vi "Create New Microservice.vi"() -> ()   [LabVIEW 2019, in "MicronToolsMenu.lvlib"]
uses:
  MicronToolsMenu.lvlib
  <vilib>/Utility/error.llb/DialogType.ctl
  <vilib>/SLL Toolkit/SLL Queued State Machine/Queue Driver/Create Queue.vi
  <vilib>/SLL Toolkit/SLL Queued State Machine/Queue Driver/Enqueue an Item to Queue.vi
  <vilib>/SLL Toolkit/SLL Queued State Machine/Queue Driver/Dequeue Queue.vi
  <vilib>/SLL Toolkit/SLL Queued State Machine/Queue Driver/Enqueue N Items.vi
  <vilib>/SLL Toolkit/SLL Queued State Machine/Queue Driver/Flush Queue.vi
  <vilib>/SLL Toolkit/SLL Queued State Machine/Queue Driver/Release Queue.vi
  <vilib>/SLL Toolkit/SLL Queued State Machine/SLL QSM.lvlib
panel:
  out "Status":string
  out "New Microservice Path Output":path
  in  "New Microservice Name":string
  in  "Root Directory":path
  in  "Create":bool
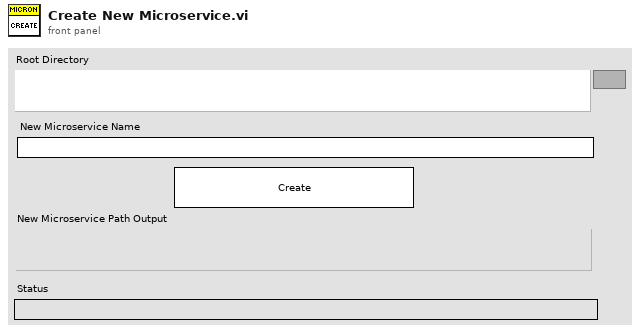
[diagram p1: front panel]
types:
  T1 = typedef "DialogType.ctl" = u16
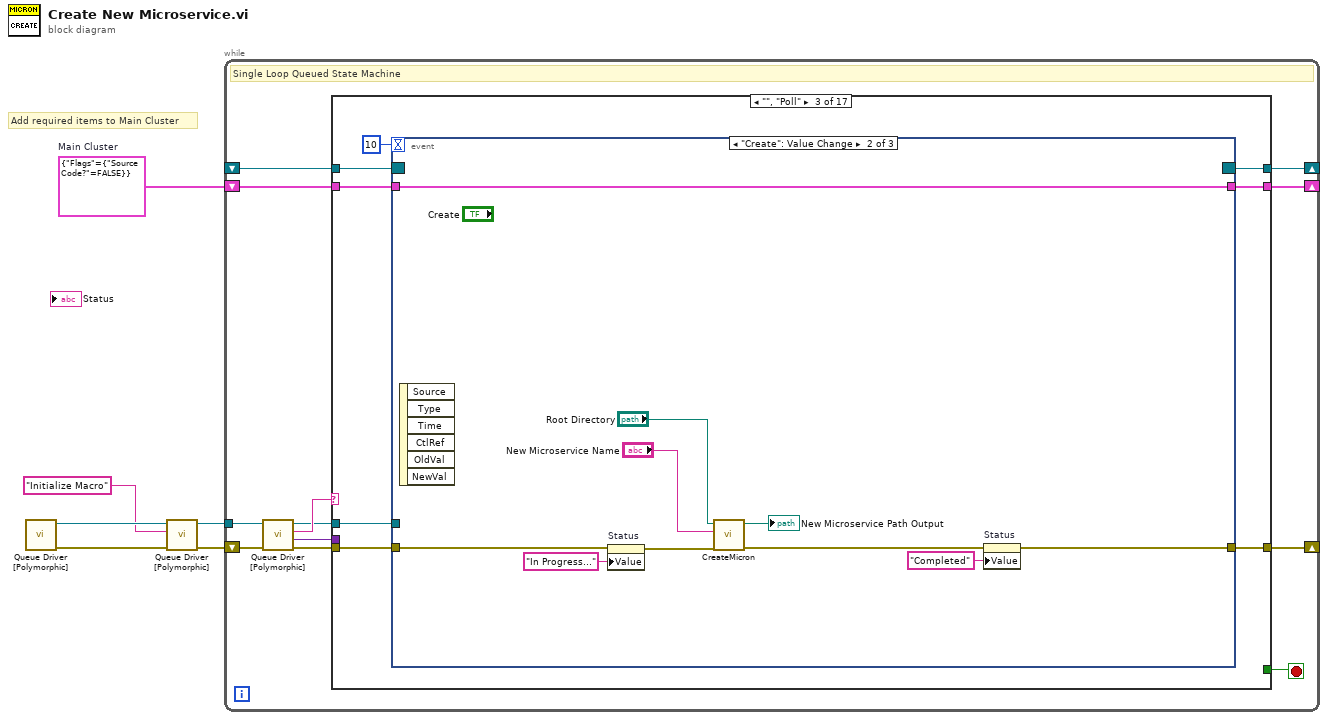
[diagram p0: block diagram]
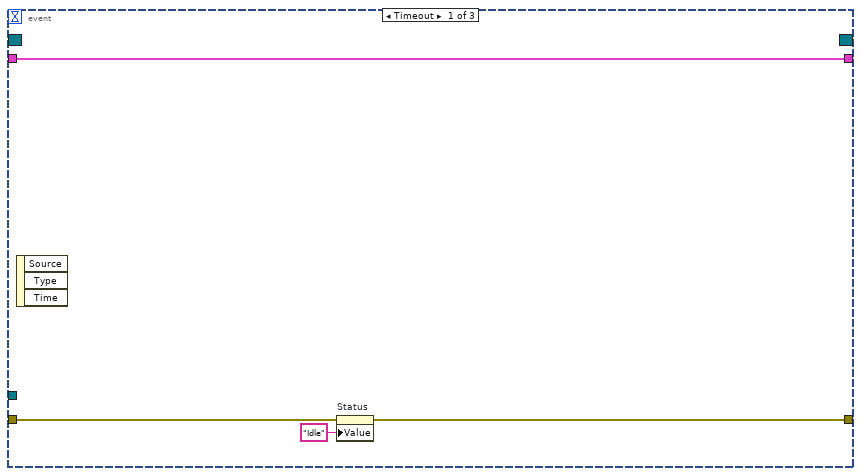
[diagram p4: hidden frame]
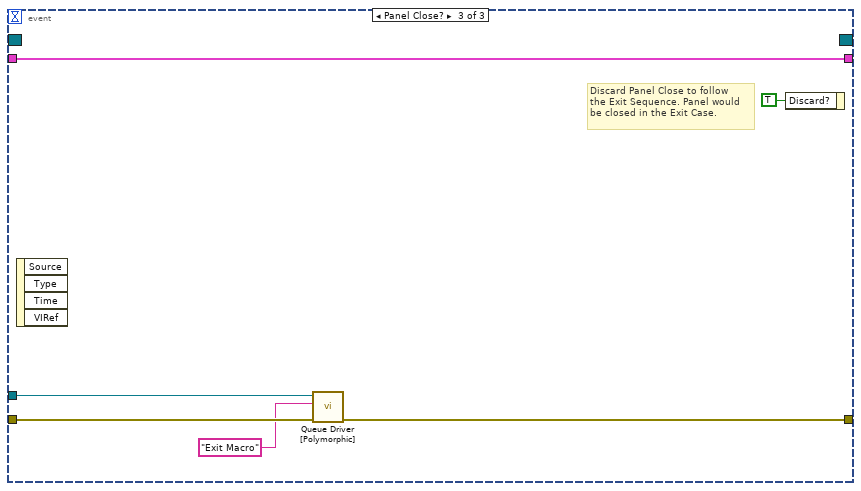
[diagram p5: hidden frame]
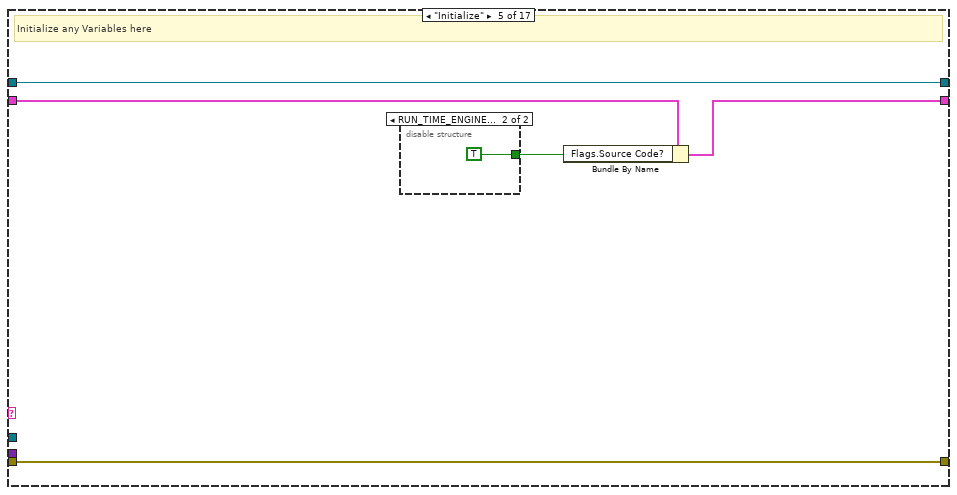
[diagram p7: hidden frame]
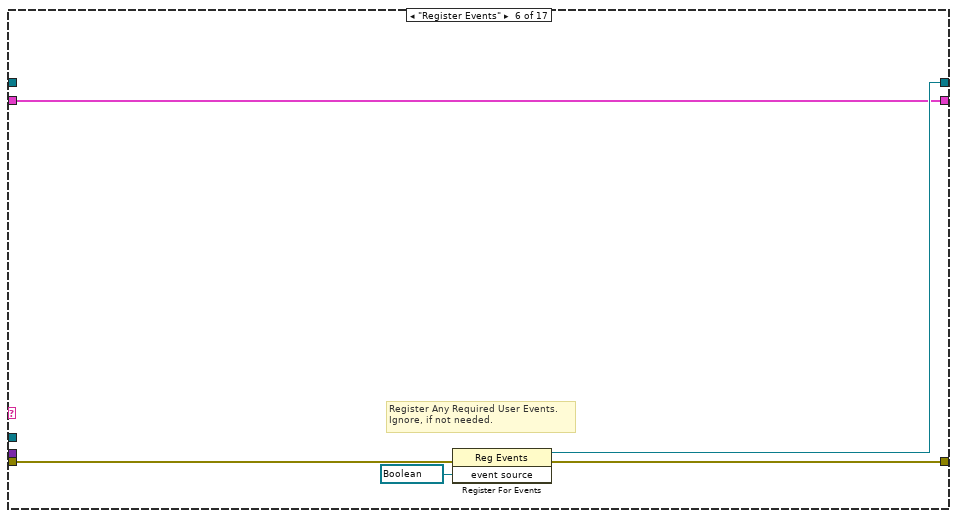
[diagram p9: hidden frame]
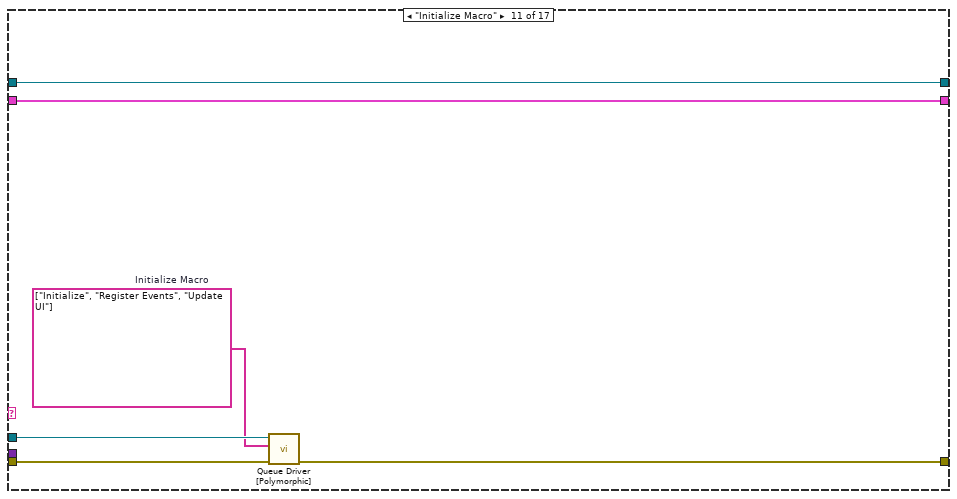
[diagram p14: hidden frame]
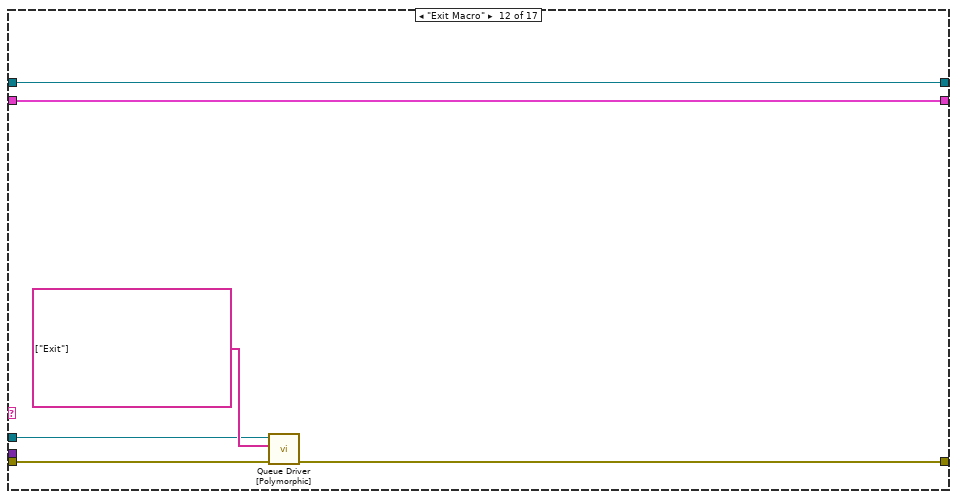
[diagram p15: hidden frame]
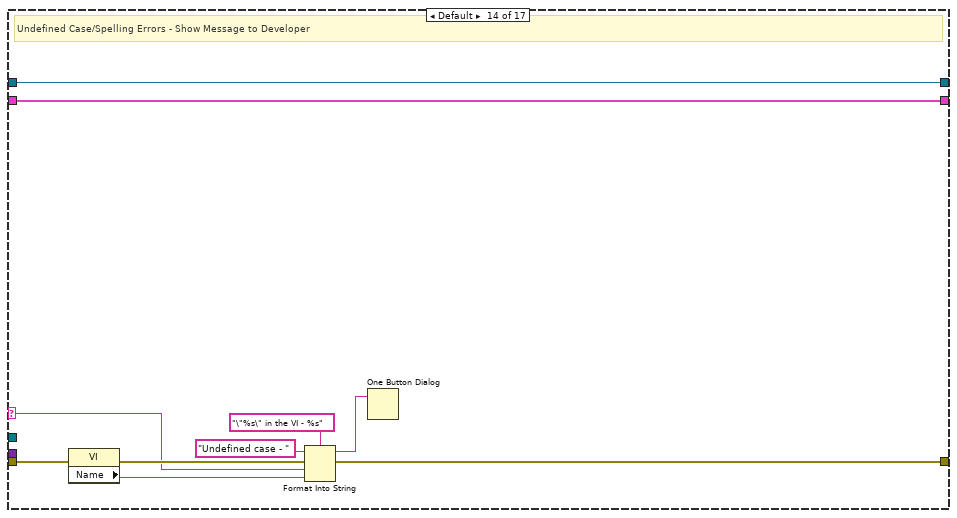
[diagram p17: hidden frame]
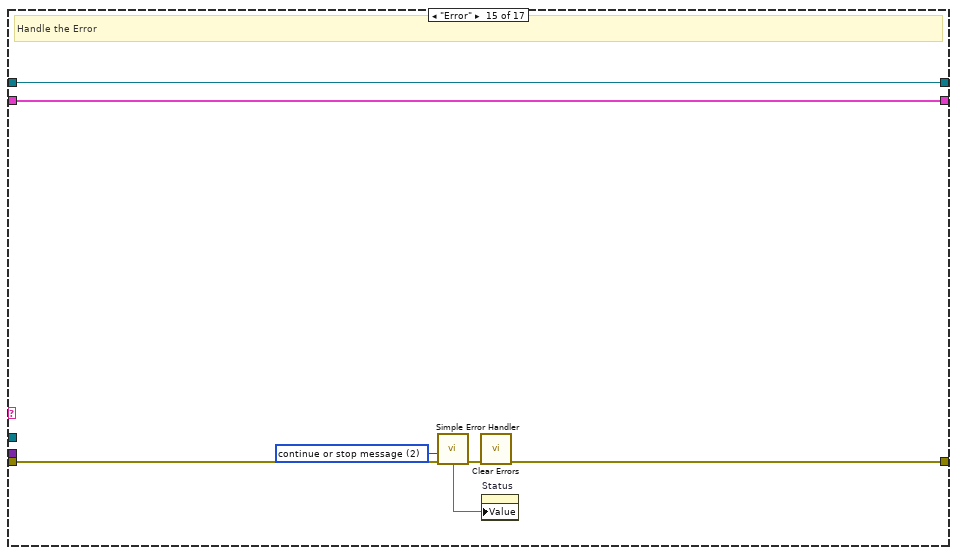
[diagram p18: hidden frame]
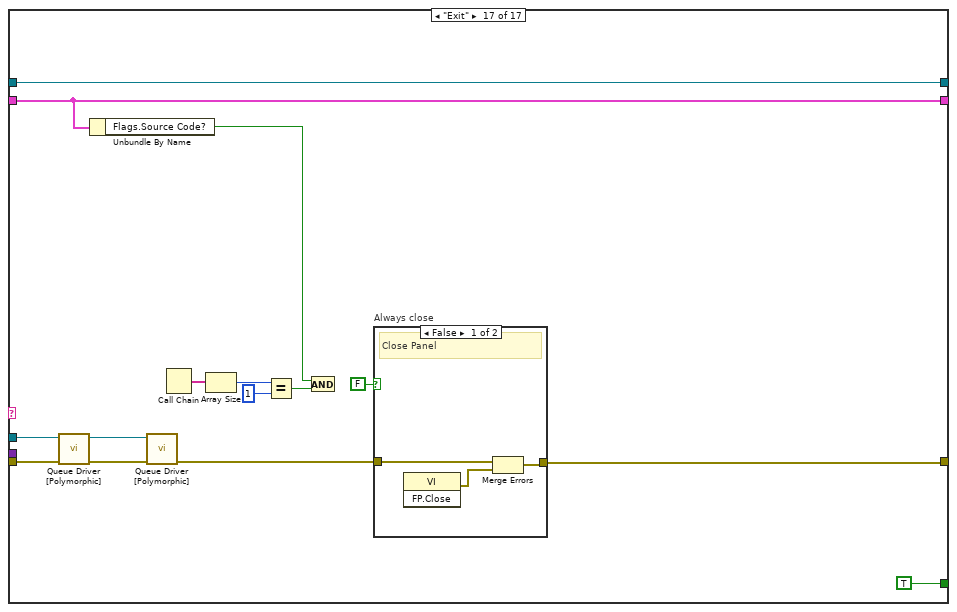
[diagram p20: hidden frame]
diagram:
  w3 = cluster{"Flags":cluster{"Source Code?":bool}} {"Flags"={"Source Code?"=FALSE}}  # Main Cluster
  # "Add required items to Main Cluster"
  n1 = call-poly <vilib>:"Queue Driver [Polymorphic].vi"() -> ("Error Out"=w1:errorcluster, "Queue Ref"=w5:refnum<queue>)  [unwired: 10 in]
  n2 = call-poly <vilib>:"Queue Driver [Polymorphic].vi"("Error In"=w1, "Item to Add"="Initialize Macro", "Queue Ref In"=w5) -> ("Error Out"=w2:errorcluster, "Queue Ref Out"=w6:refnum<queue>)  [unwired: 7 in]
  n3 = while "SLL Queued State Machine" {
    shift-right: [w16] -> _
    shift-left: w2 -> [w18]
    shift-right: [w14] -> _
    shift-left: _ -> [w13]
    shift-right: [w12] -> _
    shift-left: w3 -> [w11]
    tunnel: w6 -> [w9]
    stop <- w15 stop-if-true
    # "Single Loop Queued State Machine"
    n4 = call-poly <vilib>:"Queue Driver [Polymorphic].vi"("Error In"=w18, "Queue Ref In"=w9) -> ("Error Out"=w17:errorcluster, "Data"=w7:variant, "Dequeue"=w10:string, "Queue Ref Out"=w8:refnum<queue>)  [unwired: 6 in]
    n5 = case "QSM Case Structure" shown="\"\", \"Poll\"" w10 {
      selector: w10 -> [_ _ _ _ _ _ _ _ _ _ _ _ _ w94 _ _ _]
      tunnel: w17 -> [w21 w24 w30 w55 w60 w66 w69 w72 w75 w78 w82 w88 w93 w97 w110 w113 w126]
      tunnel: [w21 w24 w31 w55 w60 w65 w69 w72 w75 w78 w81 w87 w93 w100 w108 w113 w122] -> w16
      tunnel: [_ _ _ _ _ _ _ _ _ _ _ _ _ _ _ _ TRUE] -> w15
      tunnel: [w20 w23 w29 w54 w59 w64 w68 w71 w74 w77 w84 w90 w92 w103 w107 w112 w125] -> w14
      tunnel: w13 -> [w20 w23 w28 w54 w59 _ w68 w71 w74 w77 w84 w90 w92 w103 w107 w112 w125]
      tunnel: [w19 w22 w26 w53 w56 w63 w67 w70 w73 w76 w83 w89 w91 w102 w106 w111 w124] -> w12
      tunnel: w11 -> [w19 w22 w27 w53 w57 w63 w67 w70 w73 w76 w83 w89 w91 w102 w106 w111 w124]
      tunnel: w8 -> [_ _ w25 _ _ _ _ _ _ _ w80 w85 _ _ _ _ w116]
      tunnel: w7 -> [_ _ _ _ _ _ _ _ _ _ _ _ _ _ _ _ _]
      frame "/--------------- Read Me -----------------/" {
        # "General Purpose Queue Based State Machine for Any Use Case (main application, module, pop up message etc)\n\nAdvantages:\n1. Lean Project Code Base (dependencies are in vilib).\n2. This template can be safely used in multiple parallel running modules without any issues.\n3. This template can also be safely used even in cases where the VI is configured to be a clone, where multiple \ninstances of the VI could be executing concurrently.\n\nHow to Use:\n1. Add necessary items to the Main Cluster.\n2. Use the Polymorphic Queue Driver for doing any queue operations. \n3. Add any required user events in the \"Register Events\" case. Ignore if not needed.\n4. Use \"Macros\" section for defining any list of state calls, which could be used in multiple places. \nEx: Initialize Macro, might be needed if we need to any reinitialization."
      }
      frame "/------------------ Poll -------------------/" {
      }
      frame "", "Poll" {
        n6 = event shown="[1] \"Create\": Value Change" {
          selector: w28 -> [_ _ _]
          dyn-events: [_ _ _] -> w29
          timeout: 10 -> [_ _ _]
          tunnel: [w35 w39 w51] -> w31
          tunnel: w30 -> [w34 w42 w52]
          tunnel: w27 -> [w36 w46 w50]
          tunnel: [w36 w46 w50] -> w26
          tunnel: w25 -> [_ _ w48]
          event Timeout {
            n7 = event-data() -> ()  [unwired: 1 in, 3 out]
            n8 = property on="Status" class="Str"(error in=w34, "Value"="Idle" ("Status")) -> (error out=w35:errorcluster)  [unwired: 1 in, 1 out]
          }
          event "Create": Value Change {
            n9 = event-data() -> ()  [unwired: 1 in, 6 out]
            n10 = property on="Status" class="Str"(error in=w42, "Value"="In Progress..." ("Status")) -> (error out=w41:errorcluster)  [unwired: 1 in, 1 out]
            n11 = call "CreateMicron.vi"("error in (no error)"=w41, "New Microservice Name"="New Microservice Name", "Root Directory"="Root Directory") -> ("error out"=w40:errorcluster, "Project Path Out"=→"New Microservice Path Output":path)  [unwired: 7 in]
            n12 = property on="Status" class="Str"(error in=w40, "Value"="Completed" ("Status")) -> (error out=w39:errorcluster)  [unwired: 1 in, 1 out]
          }
          event Panel Close? {
            # "Discard Panel Close to follow\nthe Exit Sequence. Panel would\nbe closed in the Exit Case."
            n13 = event-data() -> ()  [unwired: 1 in, 4 out]
            n14 = call-poly <vilib>:"Queue Driver [Polymorphic].vi"("Error In"=w52, "Item to Add"="Exit Macro" ("Enqueue"), "Queue Ref In"=w48) -> ("Error Out"=w51:errorcluster)  [unwired: 7 in, 1 out]
            n15 = event-data("Discard?"=TRUE) -> ()  [unwired: 1 in, 1 out]
          }
        }
      }
      frame "/--------------- Initialize -----------------/" {
      }
      frame "Initialize" {
        # "Initialize any Variables here"
        n16 = disable-structure shown="RUN_TIME_ENGINE==False" {
          disable-tunnel: [_ TRUE] -> w58
          frame condition #0 {
          }
          frame condition #1 (active) {
          }
        }
        n17 = Bundle By Name(cluster=w57, "Flags.Source Code?"=w58) -> (w56:cluster{"Flags":cluster{"Source Code?":bool}})
      }
      frame "Register Events" {
        # "Register Any Required User Events. \nIgnore, if not needed."
        n18 = register-events(error in=w66, refnum<vi> refnum ("event source")) -> (reference out=w64:refnum<event-registration>, error out=w65:errorcluster)  [unwired: 1 in]
      }
      frame "/---------- Custom Case Splitter ----------/" {
      }
      frame "/-------------- User Interface --------------/" {
        # "Duplicate this case to create additional case splitters for readability"
      }
      frame "Update UI" {
        # "Update Front Panel Controls in this Case"
      }
      frame "/----------------- Macros -----------------/" {
      }
      frame "Initialize Macro" {
        w79 = string[] ["Initialize", "Register Events", "Update UI"]  # Initialize Macro
        n19 = call-poly <vilib>:"Queue Driver [Polymorphic].vi"("Error In"=w82, "Enqueue N"=w79, "Queue Ref In"=w80) -> ("Error Out"=w81:errorcluster)  [unwired: 7 in, 1 out]
      }
      frame "Exit Macro" {
        n20 = call-poly <vilib>:"Queue Driver [Polymorphic].vi"("Error In"=w88, "Enqueue N"=string[] ["Exit"], "Queue Ref In"=w85) -> ("Error Out"=w87:errorcluster)  [unwired: 7 in, 1 out]
      }
      frame "/-------------- Error Handler--------------/" {
      }
      frame Default {
        # "Undefined Case/Spelling Errors - Show Message to Developer"
        n21 = property class="VI"(error in=w97) -> (error out=w96:errorcluster, "Name"=w95:string)  [unwired: 1 in, 1 out]
        n22 = Format Into String(format string="\"%s\" in the VI - %s" ("message"), initial string="Undefined case - ", error in=w96, w94, w95) -> (resulting string=w98:string, error out=w100:errorcluster)
        n23 = One Button Dialog(message=w98) -> ()  [unwired: 1 in, 1 out]
      }
      frame "Error" {
        w105 = T1 2 items=["no dialog", "OK message", "continue or stop message", "OK message + warnings", "continue/stop + warnings"] ("type of dialog (OK msg:1)")
        # "Handle the Error"
        n24 = call <vilib>:"Simple Error Handler.vi"("type of dialog (OK msg:1)"=w105, "error in (no error)"=w110) -> ("error out"=w109:errorcluster, "message"=w104:string)  [unwired: 3 in, 3 out]
        n25 = call <vilib>:"Clear Errors.vi"("error in (no error)"=w109) -> ("error out"=w108:errorcluster)  [unwired: 5 in, 1 out]
        n26 = property on="Status" class="Str"("Value"=w104) -> ()  [unwired: 2 in, 2 out]
      }
      frame "/------------------- Exit --------------------/" {
      }
      frame "Exit" {
        n27 = call-poly <vilib>:"Queue Driver [Polymorphic].vi"("Error In"=w126, "Queue Ref In"=w116) -> ("Error Out"=w127:errorcluster, "Queue Ref Out"=w115:refnum<queue>)  [unwired: 7 in, 1 out]
        n28 = Unbundle By Name(w124) -> ("Flags.Source Code?"=w117:bool)
        n29 = call-poly <vilib>:"Queue Driver [Polymorphic].vi"("Error In"=w127, "Queue Ref In"=w115) -> ("Error Out"=w123:errorcluster)  [unwired: 9 in]
        n30 = Call Chain() -> (call chain=w121:string[])
        n31 = Array Size(array=w121) -> (size(s)=w120:i32)
        n32 = Equal?(x=w120, y=1) -> (x = y?=w118:bool)
        n33 = And(x=w117, y=w118) -> ()  [unwired: 1 out]
        n34 = case "Always close" shown="False" FALSE {
          tunnel: w123 -> [w130 w132]
          tunnel: [w131 w132] -> w122
          frame False {
            # "Close Panel"
            n35 = invoke class="VI" method="FP.Close"() -> (error out=w129:errorcluster)  [unwired: 3 in, 2 out]
            n36 = Merge Errors(w130, w129) -> (w131:errorcluster)
          }
          frame True {
            # "Do Not Close Panel"
          }
        }
      }
    }
  }
